vi "contrast converter.vi"(9 "now position":cluster{"x":dbl, "y":dbl, "degree":dbl}, 11 "contrast move array":T1[](array[typedef])) -> (1 "position out":cluster{"x":dbl, "y":dbl, "degree":dbl}, 3 "move array":T1[](array[typedef]))   [LabVIEW 2019]
uses:
  ctl/continued move array-V2.ctl
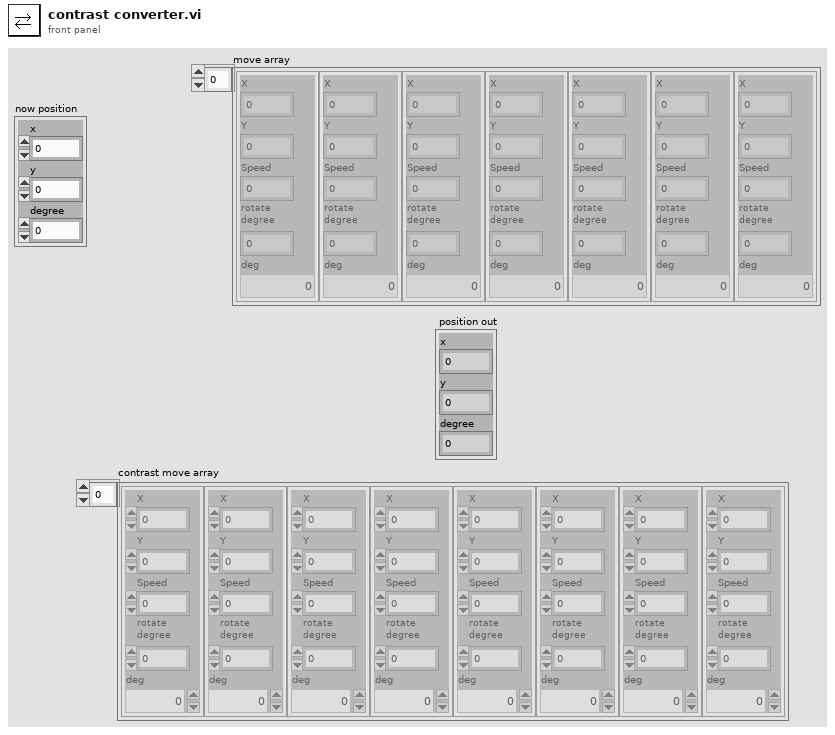
[diagram p1: front panel]
types:
  T1 = typedef "continued move array-V2.ctl" = cluster{"X":dbl, "Y":dbl, "Speed":dbl, "rotate\ndegree":dbl, "deg":dbl}
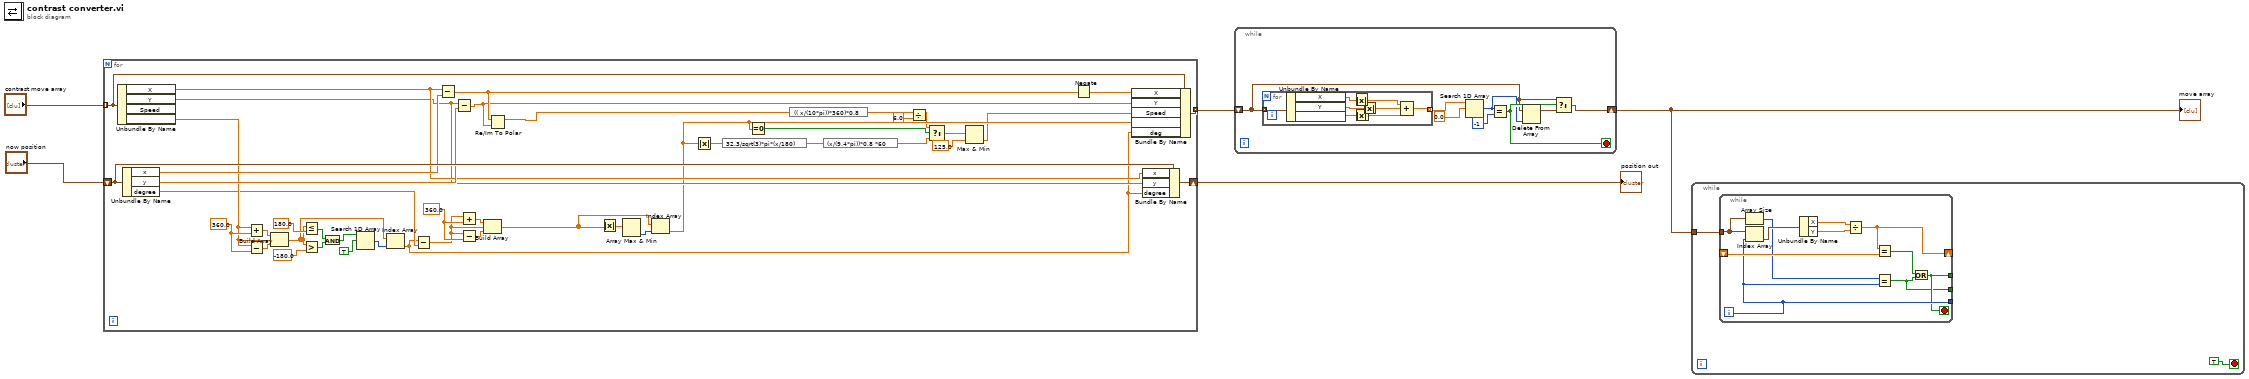
[diagram p0: block diagram]
diagram:
  n1 = for {
    tunnel: "contrast move array" -> [w44] mode=indexing
    shift-right: [w49] -> w3
    shift-left: "now position" -> [w48]
    tunnel: [w45] -> w2 mode=indexing
    w32 = 360.0
    w43 = 360.0
    n2 = Unbundle By Name(w44) -> ("X"=w23:dbl, "Y"=w22:dbl, "rotate\ndegree"=w25:dbl)  [unwired: 1 out]
    n3 = Unbundle By Name(w48) -> ("x"=w47:dbl, "y"=w46:dbl, "degree"=w24:dbl)
    n4 = Add(x=w25, y=w43) -> (x+y=w42:dbl)
    n5 = Subtract(x=w25, y=w43) -> (x-y=w41:dbl)
    n6 = Build Array(w42, w25, w41) -> (w33:dbl[])
    n7 = Less Or Equal?(x=w33, y=180.0) -> (x <= y?=w38:bool[])
    n8 = Greater?(x=w33, y=-180.0) -> (0:w37:bool[])
    n9 = And(x=w38, y=w37) -> (x .and. y?=w36:bool[])
    n10 = Search 1D Array(1D array=w36, element=TRUE) -> (index of element=w34:i32)  [unwired: 1 in]
    n11 = Index Array(array=w33, index=w34) -> (element=w10:dbl)
    n12 = Subtract(x=w10, y=w24) -> (x-y=w30:dbl)
    n13 = Subtract(x=w23, y=w47) -> (x-y=w12:dbl)
    n14 = Subtract(x=w22, y=w46) -> (x-y=w11:dbl)
    n15 = Add(x=w30, y=w32) -> (x+y=w31:dbl)
    n16 = Subtract(x=w30, y=w32) -> (x-y=w29:dbl)
    n17 = Build Array(w31, w30, w29) -> (w26:dbl[])
    n18 = Re/Im To Polar(2:w11, 3:w12) -> (1:w7:dbl)  [unwired: 1 out]
    n19 = Absolute Value(x=w26) -> (abs(x)=w28:dbl[])
    n20 = Array Max & Min(array=w28) -> (min index (indices)=w27:i32)  [unwired: 3 out]
    n21 = Index Array(array=w26, index=w27) -> (element=w20:dbl)
    n22 = Absolute Value(x=w20) -> (abs(x)=w16:dbl)
    n23 = expression code="32.3/sqrt(3)*pi*(x/180)"(w16) -> (w21:dbl)
    n24 = Equal To 0?(x=w20) -> (x = 0?=w19:bool)
    n25 = expression code="(( x/(10*pi))*360)*0.8"(w7) -> (w18:dbl)
    n26 = expression code="(x/(9.4*pi))*0.8 *60"(w21) -> (w17:dbl)
    n27 = Divide(x=w18, y=6.0) -> (x/y=w9:dbl)
    n28 = Select(t=w9, s=w19, f=w17) -> (s? t:f=w15:dbl)
    n29 = Max & Min(x=w15, y=125.0) -> (min(x,y)=w13:dbl)  [unwired: 1 out]
    n30 = Negate(x=w12) -> (-x=w6:dbl)
    n31 = Bundle By Name(cluster=w44, "X"=w6, "Y"=w11, "Speed"=w13, "rotate\ndegree"=w20, "deg"=w10) -> (w45:T1)
    n32 = Bundle By Name(cluster=w48, "x"=w23, "y"=w22, "degree"=w10) -> (w49:cluster{"x":dbl, "y":dbl, "degree":dbl})
  }
  "position out" <- w3
  n33 = while {
    shift-right: [w53] -> w1
    shift-left: w2 -> [w52]
    stop <- w54 stop-if-true
    n34 = for {
      tunnel: w52 -> [w65] mode=indexing
      tunnel: [w58] -> w57 mode=indexing
      n35 = Unbundle By Name(w65) -> ("X"=w64:dbl, "Y"=w63:dbl, "rotate\ndegree"=w62:dbl)
      n36 = Absolute Value(x=w64) -> (abs(x)=w60:dbl)
      n37 = Absolute Value(x=w62) -> (abs(x)=w59:dbl)
      n38 = Absolute Value(x=w63) -> (abs(x)=w61:dbl)
      n39 = Compound Arithmetic op=ADD(w60, w61, w59) -> (w58:dbl)
    }
    n40 = Search 1D Array(1D array=w57, element=0.0) -> (index of element=w50:i32)  [unwired: 1 in]
    n41 = Equal?(x=w50, y=-1) -> (x = y?=w54:bool)
    n42 = Delete From Array(array=w52, index=w50) -> (array with subset deleted=w51:T1[])  [unwired: 1 in, 1 out]
    n43 = Select(t=w52, s=w54, f=w51) -> (s? t:f=w53:T1[])
  }
  "move array" <- w1
  n44 = while {
    tunnel: w1 -> [w67]
    stop <- TRUE stop-if-true
    n45 = while {
      tunnel: w67 -> [w73]
      shift-right: [w76] -> _
      shift-left: _ -> [w75]
      tunnel: [w71] -> _
      tunnel: [w70] -> _
      tunnel: [w69] -> _
      i -> [w71]
      stop <- w70 stop-if-true
      n46 = Array Size(array=w73) -> (size(s)=w72:i32)
      n47 = Index Array(array=w73, index=w71) -> (element=w74:T1)
      n48 = Unbundle By Name(w74) -> ("X"=w77:dbl, "Y"=w78:dbl)
      n49 = Divide(x=w77, y=w78) -> (x/y=w76:dbl)
      n50 = Equal?(x=w76, y=w75) -> (x = y?=w68:bool)
      n51 = Equal?(x=w72, y=w71) -> (x = y?=w69:bool)
      n52 = Or(x=w68, y=w69) -> (x .or. y?=w70:bool)
    }
  }
